vi "Interpolator_Yuhe.vi"(10 "interpolation distance":dbl, 11 "Array in":cluster{"X":dbl, "Y":dbl}[](array[cluster])) -> (3 "Array out":cluster{"X":dbl, "Y":dbl}[](array[cluster]))   [LabVIEW 2016]
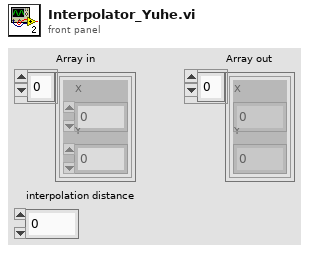
[diagram p1: front panel]
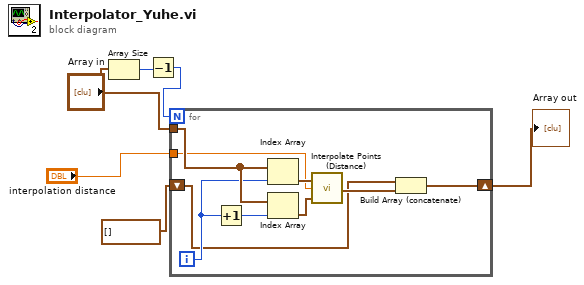
[diagram p0: block diagram]
diagram:
  n1 = Array Size(array="Array in") -> (size(s)=w1:i32)
  n2 = Decrement(x=w1) -> (x-1=w2:i32)
  n3 = for {
    N: w2 -> [_]
    tunnel: "Array in" -> [w15]
    tunnel: "interpolation distance" -> [w10]
    shift-right: [w8] -> w5
    shift-left: cluster{"X":dbl, "Y":dbl}[] [] -> [w7]
    i -> [w14]
    n4 = Increment(x=w14) -> (x+1=w13:i32)
    n5 = Index Array(array=w15, index=w14) -> (element=w12:cluster{"X":dbl, "Y":dbl})
    n6 = Index Array(array=w15, index=w13) -> (element=w11:cluster{"X":dbl, "Y":dbl})
    n7 = call "Interpolate Points (Distance).vi"("End Point"=w11, "Distance between Points"=w10, "Start Point"=w12) -> ("Output Point Array"=w9:cluster{"X":dbl, "Y":dbl}[])
    n8 = Build Array (concatenate)(w7, w9) -> (w8:cluster{"X":dbl, "Y":dbl}[])
  }
  "Array out" <- w5
